vi "FPGA_laser_control.vi"() -> ()   [LabVIEW 2015]
uses:
  <vilib>/rvi/eio/common/nirviEmuTemplateMethod_errors.vi
  <vilib>/eio/EIONode/EIONode.xnode
panel:
  in  "488":sgl
  in  "405":sgl
  in  "640":sgl
  in  "561":sgl
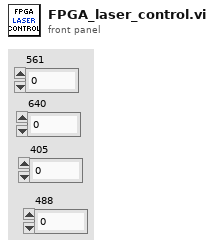
[diagram p1: front panel]
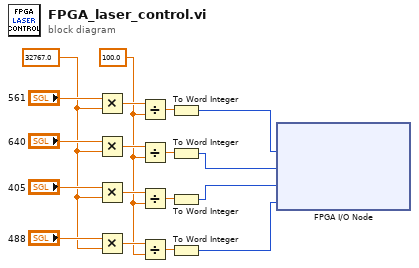
[diagram p0: block diagram]
diagram:
  w2 = sgl 100.0
  w3 = sgl 32767.0
  n1 = Multiply(x="561", y=w3) -> (x*y=w17:sgl)
  n2 = Multiply(x="640", y=w3) -> (x*y=w13:sgl)
  n3 = Multiply(x="405", y=w3) -> (x*y=w9:sgl)
  n4 = Multiply(x="488", y=w3) -> (x*y=w5:sgl)
  n5 = Divide(x=w17, y=w2) -> (x/y=w16:sgl)
  n6 = Divide(x=w13, y=w2) -> (x/y=w14:sgl)
  n7 = Divide(x=w9, y=w2) -> (x/y=w8:sgl)
  n8 = Divide(x=w5, y=w2) -> (x/y=w6:sgl)
  n9 = To Word Integer(number=w16) -> (16bit integer=w15:i16)
  n10 = To Word Integer(number=w14) -> (16bit integer=w11:i16)
  n11 = To Word Integer(number=w8) -> (16bit integer=w7:i16)
  n12 = To Word Integer(number=w6) -> (16bit integer=w1:i16)
  n13 = xnode "FPGA I/O Node"("Connector0/AO0"=w15, "Connector0/AO1"=w11, "Connector0/AO2"=w7, "Connector0/AO3"=w1) -> ()  [unwired: 4 in, 4 out]
